vi "Inspect Map.vi"(9 "Fault":errorcluster, 10 "Device":string, 11 "Fault map in":T1) -> (1 "Log Record":string, 3 "Fault Map out":T1)   [LabVIEW 2023, in "Fault Monitor.lvlib" / "Fault Monitor.lvclass"]
uses:
  Library/Fault Monitor.lvclass
  Custom Controls/Fault Map.ctl
  <vilib>/Utility/miscctls.llb/LVMapReplaceAction.ctl
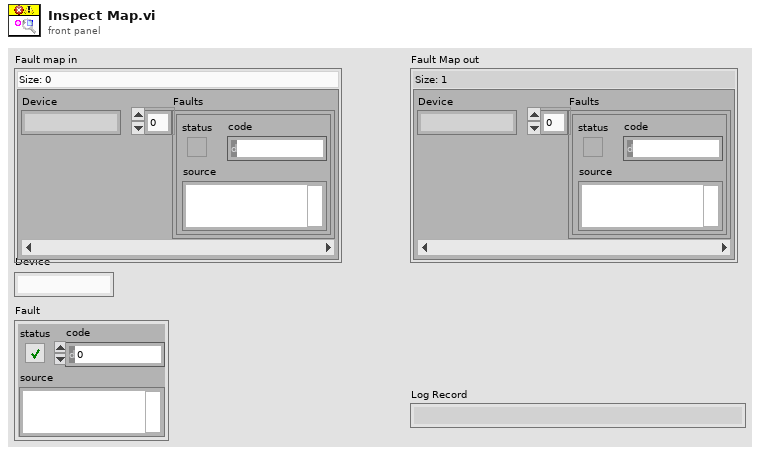
[diagram p1: front panel]
types:
  T1 = typedef "Fault Monitor.lvlib/Fault Monitor.lvclass/Fault Map.ctl" = map{string, errorcluster[]}
  T2 = typedef "LVMapReplaceAction.ctl" = enum32{"Modify Entry only if found", "Add or Modify Entry", "Delete Entry"}
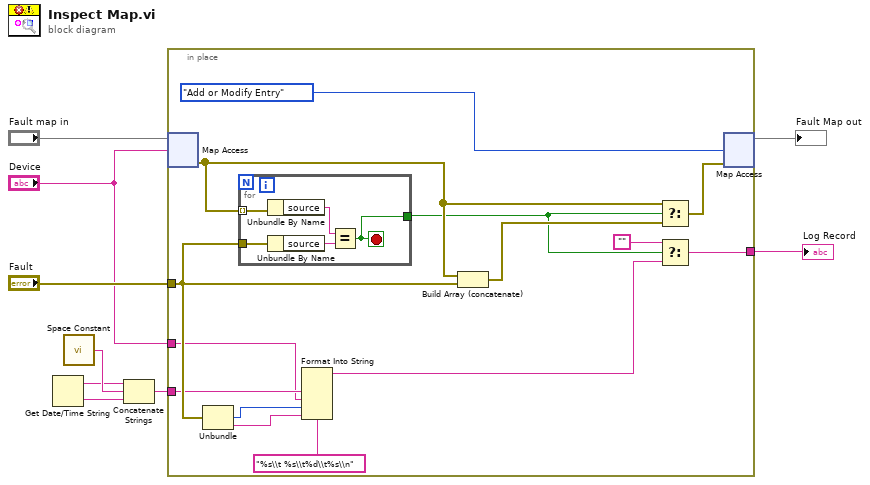
[diagram p0: block diagram]
diagram:
  n1 = Get Date/Time String() -> (date string=w6:string, time string=w5:string)  [unwired: 3 in]
  n2 = call <vilib>:"Space Constant.vi"() -> ("String"=w7:string)
  n3 = Concatenate Strings(w6, w7, w5) -> (w3:string)
  n4 = in-place {
    in-place-border: "Fault" -> [w17]
    in-place-border: w3 -> [w15]
    in-place-border: "Device" -> [w14]
    in-place-border: [w10] -> w1
    n5 = in-place-map #1("Fault map in", "Device") -> (w22:errorcluster[])  [unwired: 1 in, 1 out]
    n6 = Unbundle(w17) -> ("code"=w18:i32, "source"=w19:string)  [unwired: 1 out]
    n7 = for {
      tunnel: w22 -> [w27] mode=indexing
      tunnel: w17 -> [w28]
      tunnel: [w24] -> w13
      stop <- w24 stop-if-true
      n8 = Unbundle By Name(w27) -> ("source"=w25:string)
      n9 = Unbundle By Name(w28) -> ("source"=w26:string)
      n10 = Equal?(x=w25, y=w26) -> (x = y?=w24:bool)
    }
    n11 = Format Into String(format string="%s\\t %s\\t%d\\t%s\\n", w15, w14, w18, w19) -> (resulting string=w12:string)  [unwired: 2 in, 1 out]
    n12 = Build Array (concatenate)(w22, w17) -> (w21:errorcluster[])
    n13 = Select(t=w22, s=w13, f=w21) -> (s? t:f=w20:errorcluster[])
    n14 = Select(t="", s=w13, f=w12) -> (s? t:f=w10:string)
    n15 = in-place-map #1(w20, LVMapReplaceAction."Add or Modify Entry" ("action")) -> (→"Fault Map out":T1)  [unwired: 2 out]
  }
  "Log Record" <- w1
